vi "StraightDriveSimple.vi"(5 "Straightening PID gains":T1={"proportional gain (Kc)"=1.0, "integral time (Ti, min)"=0.01, "derivative time (Td, min)"=0.0} {"derivative time (Td, min)" format="%.3f"; "integral time (Ti, min)" format="%.3f"; "proportional gain (Kc)" format="%.3f"}, 6 "Speed":dbl format="%.2f", 7 "Speed PID gains":T1={"proportional gain (Kc)"=1.0, "integral time (Ti, min)"=0.01, "derivative time (Td, min)"=0.0} {"derivative time (Td, min)" format="%.3f"; "integral time (Ti, min)" format="%.3f"; "proportional gain (Kc)" format="%.3f"}, 9 "Tolerance [Dead Band]":dbl format="%.2f", 11 "Distance to move":dbl format="%.2f") -> ()   [LabVIEW 2012]
uses:
  <vilib>/Rock Robotics/WPI/RobotDrive/WPI_RobotDriveGetSetRefNum.vi
  <vilib>/addons/control/pid/pid.llb/PID (DBL).vi
  <vilib>/addons/control/pid/NI_PID_pid.lvlib
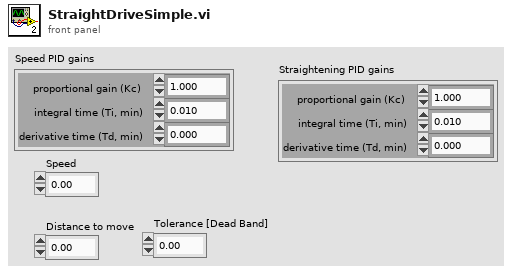
[diagram p1: front panel]
types:
  T1 = cluster{"proportional gain (Kc)":dbl, "integral time (Ti, min)":dbl, "derivative time (Td, min)":dbl}
  T2 = typedef "WPI_EncoderDevRef.ctl" = cluster{"DevStatus":errorcluster, "EncoderIndex":T3, "CounterIndex":T4, "DistancePerCount":dbl, "Decoding Type":T5}
  T3 = typedef "FPGA_EncoderIdx.ctl" = enum8{"Enc 0", "Enc 1", "Enc 2", "Enc 3", "Invalid"}
  T4 = typedef "FPGA_CounterCtrSystemIndex.ctl" = enum8{"Ctr 0", "Ctr 1", "Ctr 2", "Ctr 3", "Ctr 4", "Ctr 5", "Ctr 6", "Ctr 7", "Invalid"}
  T5 = typedef "WPI_EncoderType.ctl" = enum16{"1x", "2x", "4x"}
  T6 = typedef "WPI_RobotDriveDevRef.ctl" = cluster{"DevStatus":errorcluster, "Motors[]":T7[], "Square Inputs":bool, "Max Output":dbl, "Isochronous":bool}
  T7 = typedef "WPI_MotorControlDeviceRef.ctl" = cluster{"DeviceStatus":errorcluster, "Type":enum16{"PWM", "CAN"}, "PWM":cluster{"Digital Module":T8, "PWM Channel":T9, "DeadBand":T10}, "CAN":cluster{"Device Number":u8, "Control Mode":T11, "Semaphore":T12, "Max Vout":dbl}, "Invert":bool, "TransformRef":T13, "InvTransformRef":T13}
  T8 = typedef "FPGA_TypedefDigitalModule.ctl" = enum16{"Digital Module 1", "Digital Module 2"}
  T9 = typedef "FPGA_DIOPWMChannel.ctl" = enum8{"PWM 1", "PWM 2", "PWM 3", "PWM 4", "PWM 5", "PWM 6", "PWM 7", "PWM 8", "PWM 9", "PWM 10", "Invalid"}
  T10 = typedef "WPI_PWMDeadband.ctl" = cluster{"Name":string, "maxPositivePwm":i32, "minPositivePwm":i32, "centerPwm":i32, "maxNegativePwm":i32, "minNegativePwm":i32, "angularRange":u16}
  T11 = typedef "WPI_CANJaguar_ControlMode.ctl" = enum8{"Percent VBus", "Current", "Speed", "Position", "Voltage"}
  T12 = typedef "Semaphore RefNum" = refnum<k1>
  T13 = typedef "WPI_PWMTransform_ConPane.ctl" = refnum<vi>
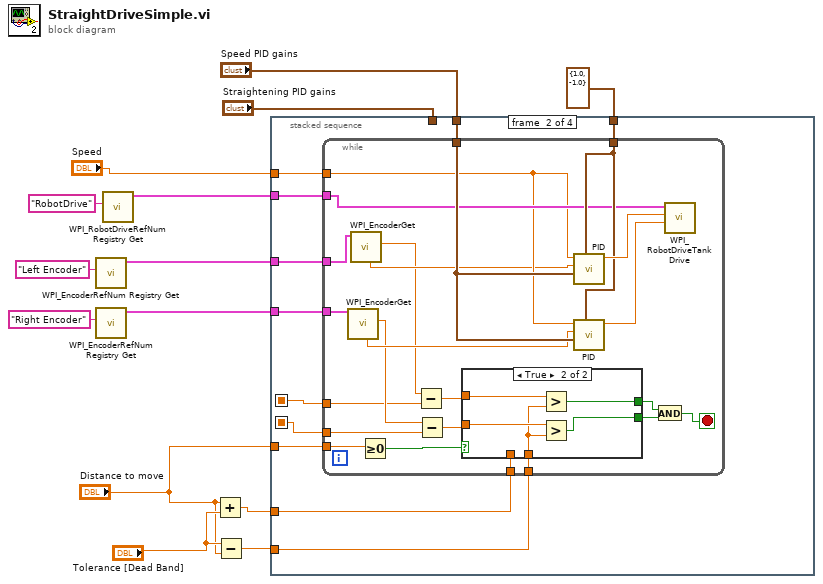
[diagram p0: block diagram]
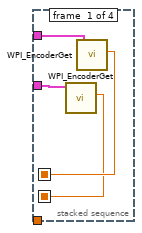
[diagram p2: hidden frame]
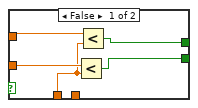
[diagram p3: hidden frame]
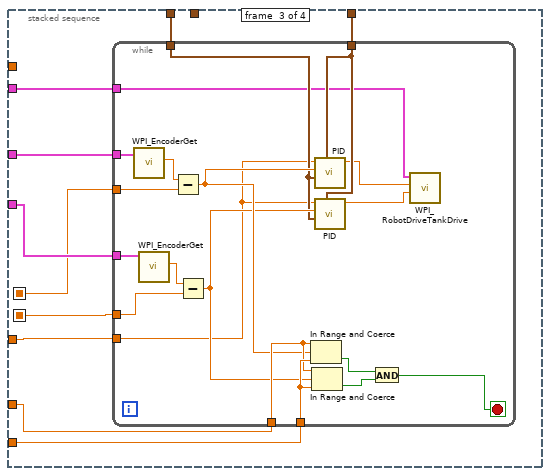
[diagram p4: hidden frame]
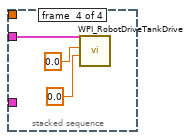
[diagram p5: hidden frame]
diagram:
  n1 = call <vilib>:"WPI_EncoderRefNum Registry Get.vi"("refnum name"="Left Encoder") -> ("EncoderDevRef"=w10:T2)  [unwired: 9 in, 1 out]
  n2 = call <vilib>:"WPI_EncoderRefNum Registry Get.vi"("refnum name"="Right Encoder") -> ("EncoderDevRef"=w9:T2)  [unwired: 9 in, 1 out]
  n3 = call <vilib>:"WPI_RobotDriveRefNum Registry Get.vi"("refnum name"="RobotDrive") -> ("RobotDriveDevRef"=w6:T6)  [unwired: 9 in, 1 out]
  n4 = Add(x="Distance to move", y="Tolerance [Dead Band]") -> (x+y=w3:dbl)
  n5 = Subtract(x="Tolerance [Dead Band]", y="Distance to move") -> (x-y=w4:dbl)
  n6 = stacked-sequence {
    seq-local: [w16 _ _ _] -> [_ w29 w70 _]
    seq-local: [w15 _ _ _] -> [_ w28 w69 _]
    tunnel: "Speed PID gains" -> [_ w23 _ _]
    tunnel: "Speed" -> [_ w22 _ _]
    tunnel: w10 -> [w17 w27 w72 _]
    tunnel: w9 -> [w18 w26 w71 _]
    tunnel: cluster{"output high":dbl, "output low":dbl} {"output high"=1.0, "output low"=-1.0} ("output range") -> [_ w24 w66 _]
    tunnel: w6 -> [_ w25 w63 w94]
    tunnel: w4 -> [_ w20 w68 _]
    tunnel: w3 -> [_ w21 w67 _]
    tunnel: "Distance to move" -> [_ w19 w64 _]
    tunnel: "Straightening PID gains" -> [_ _ w65 _]
    frame #0 {
      n7 = call <vilib>:"WPI_EncoderGet.vi"("EncoderDevRef"=w18) -> ("Distance"=w15:dbl)  [unwired: 5 in, 5 out]
      n8 = call <vilib>:"WPI_EncoderGet.vi"("EncoderDevRef"=w17) -> ("Distance"=w16:dbl)  [unwired: 5 in, 5 out]
    }
    frame #1 {
      n9 = while {
        tunnel: w23 -> [w52]
        tunnel: w22 -> [w45]
        tunnel: w24 -> [w49]
        tunnel: w25 -> [w47]
        tunnel: w29 -> [w36]
        tunnel: w28 -> [w35]
        tunnel: w27 -> [w34]
        tunnel: w26 -> [w33]
        tunnel: w21 -> [w32]
        tunnel: w20 -> [w31]
        tunnel: w19 -> [w30]
        stop <- w48 stop-if-true
        n10 = call <vilib>:"WPI_EncoderGet.vi"("EncoderDevRef"=w33) -> ("Distance"=w38:dbl, "Rate"=w43:dbl)  [unwired: 5 in, 4 out]
        n11 = call <vilib>:"WPI_EncoderGet.vi"("EncoderDevRef"=w34) -> ("Distance"=w40:dbl, "Rate"=w44:dbl)  [unwired: 5 in, 4 out]
        n12 = Greater Or Equal To 0?(x=w30) -> (x >= 0?=w46:bool)
        n13 = Subtract(x=w40, y=w36) -> (x-y=w39:dbl)
        n14 = Subtract(x=w38, y=w35) -> (x-y=w37:dbl)
        n15 = case shown="True" w46 {
          tunnel: w37 -> [w56 w61]
          tunnel: w39 -> [w57 w62]
          tunnel: [w55 w60] -> w42
          tunnel: [w54 w59] -> w41
          tunnel: w32 -> [w53 _]
          tunnel: w31 -> [_ w58]
          frame False {
            n16 = Less?(x=w56, y=w53) -> (x < y?=w55:bool)
            n17 = Less?(x=w57, y=w53) -> (x < y?=w54:bool)
          }
          frame True {
            n18 = Greater?(x=w62, y=w58) -> (0:w59:bool)
            n19 = Greater?(x=w61, y=w58) -> (0:w60:bool)
          }
        }
        n20 = call-poly <vilib>:"PID.vi"("output range"=w49, "PID gains"=w52, "process variable"=w44, "setpoint"=w45) -> ("output"=w51:dbl)  [unwired: 6 in, 1 out]
        n21 = call-poly <vilib>:"PID.vi"("output range"=w49, "PID gains"=w52, "process variable"=w43, "setpoint"=w45) -> ("output"=w50:dbl)  [unwired: 6 in, 1 out]
        n22 = And(x=w41, y=w42) -> (x .and. y?=w48:bool)
        n23 = call <vilib>:"WPI_RobotDriveTankDrive.vi"("Right axis value"=w50, "Left axis value"=w51, "RobotDriveDevRef"=w47) -> ()  [unwired: 6 in, 3 out]
      }
    }
    frame #2 {
      n24 = while {
        tunnel: w72 -> [w89]
        tunnel: w71 -> [w83]
        tunnel: w70 -> [w86]
        tunnel: w69 -> [w84]
        tunnel: w68 -> [w91]
        tunnel: w67 -> [w90]
        tunnel: w66 -> [w81]
        tunnel: w65 -> [w80]
        tunnel: w64 -> [w76]
        tunnel: w63 -> [w73]
        stop <- w77 stop-if-true
        n25 = call <vilib>:"WPI_EncoderGet.vi"("EncoderDevRef"=w89) -> ("Distance"=w88:dbl)  [unwired: 5 in, 5 out]
        n26 = call <vilib>:"WPI_EncoderGet.vi"("EncoderDevRef"=w83) -> ("Distance"=w85:dbl)  [unwired: 5 in, 5 out]
        n27 = Subtract(x=w88, y=w86) -> (x-y=w87:dbl)
        n28 = Subtract(x=w85, y=w84) -> (x-y=w82:dbl)
        n29 = In Range and Coerce(upper limit=w90, x=w87, lower limit=w91) -> (In Range?=w79:bool)  [unwired: 1 out]
        n30 = In Range and Coerce(upper limit=w90, x=w82, lower limit=w91) -> (In Range?=w78:bool)  [unwired: 1 out]
        n31 = call-poly <vilib>:"PID.vi"("output range"=w81, "PID gains"=w80, "process variable"=w87, "setpoint"=w76) -> ("output"=w74:dbl)  [unwired: 6 in, 1 out]
        n32 = call-poly <vilib>:"PID.vi"("output range"=w81, "PID gains"=w80, "process variable"=w82, "setpoint"=w76) -> ("output"=w75:dbl)  [unwired: 6 in, 1 out]
        n33 = And(x=w79, y=w78) -> (x .and. y?=w77:bool)
        n34 = call <vilib>:"WPI_RobotDriveTankDrive.vi"("Right axis value"=w75, "Left axis value"=w74, "RobotDriveDevRef"=w73) -> ()  [unwired: 6 in, 3 out]
      }
    }
    frame #3 {
      n35 = call <vilib>:"WPI_RobotDriveTankDrive.vi"("Right axis value"=0.0, "Left axis value"=0.0, "RobotDriveDevRef"=w94) -> ()  [unwired: 6 in, 3 out]
    }
  }
